vi "Begin.vi"() -> (0 "error out":errorcluster)   [LabVIEW 2014]
doc: "Called before other user functions, this VI is expected to open initial I/O refnums, load in file data, and do all program initialization. Notice that the <B>error out</B> terminal is simply used for data flow. Wiring it to other structures or subVIs ensures that this VI runs first."
uses:
  <vilib>/Rock Robotics/SystemInterfaces/DIO/FPGA_DIOPWMChannel.ctl
  <vilib>/Rock Robotics/WPI/SafetyOutput/WPI_SafetyOutputConfigMenu.ctl
  <vilib>/Rock Robotics/WPI/DriverStation/WPI_DriverStationRobotMode2.ctl
  <vilib>/Rock Robotics/WPI/Joystick/WPI_JoystickDeviceEnum.ctl
  <vilib>/Rock Robotics/SystemInterfaces/AI/FPGA_AIChannel.ctl
  <vilib>/Rock Robotics/SystemInterfaces/AI/FPGA_AIGyroChannel.ctl
  <vilib>/Rock Robotics/SystemInterfaces/DIO/FPGA_DIOChannel.ctl
  <vilib>/Rock Robotics/SystemInterfaces/DIO/FPGA_DIORelayChannel.ctl
  Robot Global Data.vi
  <vilib>/Rock Robotics/WPI/RobotDrive/WPI_RobotDriveOpen4MotorWithVictor.vi
  <vilib>/Rock Robotics/WPI/MotorControl/WPI_MotorControlOpen Victor.vi
  Events.vi
  Robot Global ref.vi
  AutonVars.vi
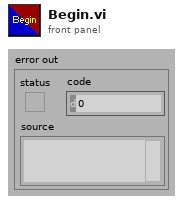
[diagram p1: front panel]
types:
  T1 = typedef "FPGA_DIORelayChannel.ctl" = enum8{"Relay 1", "Relay 2", "Relay 3", "Relay 4", "Relay 5", "Relay 6", "Relay 7", "Relay 8", "Invalid"}
  T2 = typedef "FPGA_DIOChannel.ctl" = enum8{"DIO 1", "DIO 2", "DIO 3", "DIO 4", "DIO 5", "DIO 6", "DIO 7", "DIO 8", "DIO 9", "DIO 10", "DIO 11", "DIO 12", "DIO 13", "DIO 14", "Invalid"}
  T3 = typedef "FPGA_DIOPWMChannel.ctl" = enum8{"PWM 1", "PWM 2", "PWM 3", "PWM 4", "PWM 5", "PWM 6", "PWM 7", "PWM 8", "PWM 9", "PWM 10", "Invalid"}
  T4 = typedef "FPGA_AIGyroChannel.ctl" = enum8{"AI 1", "AI 2", "Invalid"}
  T5 = typedef "WPI_JoystickDeviceEnum.ctl" = enum16{"USB 0", "USB 1", "USB 2", "USB 3", "USB 4", "USB 5"}
  T6 = typedef "FPGA_AIChannel.ctl" = enum8{"AI 1", "AI 2", "AI 3", "AI 4", "AI 5", "AI 6", "AI 7", "AI 8", "Invalid"}
  T7 = typedef "WPI_DriverStationRobotMode2.ctl" = enum16{"Autonomous Disabled", "Autonomous Enabled", "Teleop Disabled", "Teleop Enabled", "Disconnected", "Finish", "Test Disabled", "Test Enabled"}
  T8 = typedef "WPI_SafetyOutputConfigMenu.ctl" = enum16{"Enable", "Disable"}
  T9 = typedef "WPI_RobotDriveDevRef.ctl" = cluster{"DevStatus":errorcluster, "Motors[]":T10[], "Square Inputs":bool, "Max Output":dbl}
  T10 = typedef "WPI_MotorControlDeviceRef.ctl" = cluster{"DeviceStatus":errorcluster, "Type":enum16{"PWM", "CAN"}, "PWM":cluster{"Digital Module":T11, "PWM Channel":T3, "DeadBand":T12}, "CAN":cluster{"Device Number":u8, "Control Mode":T13, "Semaphore":T14, "Max Vout":dbl}, "Invert":bool, "TransformRef":T15, "InvTransformRef":T15}
  T11 = typedef "FPGA_TypedefDigitalModule.ctl" = enum16{"Digital Module 1", "Digital Module 2"}
  T12 = typedef "WPI_PWMDeadband.ctl" = cluster{"Name":string, "maxPositivePwm":i32, "minPositivePwm":i32, "centerPwm":i32, "maxNegativePwm":i32, "minNegativePwm":i32, "angularRange":u16}
  T13 = typedef "WPI_CANJaguar_ControlMode.ctl" = enum8{"Percent VBus", "Current", "Speed", "Position", "Voltage"}
  T14 = typedef "Semaphore RefNum" = refnum<k1>
  T15 = typedef "WPI_PWMTransform_ConPane.ctl" = refnum<vi>
  T16 = typedef "WPI_DigitalInputDevRef.ctl" = cluster{"DevStatus":errorcluster, "DIO Channel":T2, "Digital Module":T11}
  T17 = typedef "WPI_GyroDevRef.ctl" = cluster{"DevStatus":errorcluster, "Analog Module":T18, "Analog Channel":T6, "Offset":dbl, "Gain (VoltsPerDegree/Second)":dbl}
  T18 = typedef "FPGA_TypedefAnalogModule.ctl" = enum16{"Analog Module 1", "Analog Module 2"}
  T19 = typedef "WPI_ServoDeviceRef.ctl" = cluster{"DeviceStatus":errorcluster, "Digital Module":T11, "PWM Channel":T3, "DeadBand":T12}
  T20 = typedef "WPI_JoystickDevRef.ctl" = cluster{"Device":T5}
  T21 = typedef "WPI_AnalogChannelDevRef.ctl" = cluster{"DevStatus":errorcluster, "Analog Module":T18, "Analog Channel":T6}
  T22 = typedef "WPI_RelayDevRef.ctl" = cluster{"DevStatus":errorcluster, "Relay Channel":T1, "Digital Module":T11, "Relay Direction":T23}
  T23 = typedef "WPI_RelayDirection.ctl" = enum16{"Both directions", "Forward only", "Reverse only"}
  T24 = typedef "Eventgrab.ctl" = cluster{"Grab":bool, "GroundPass":bool, "Test Aqaure":dbl, "Shoulder up or down?":bool, "Auton drag":bool}
  T25 = typedef "Robot Global ref.ctl" = cluster{"Joysticks":cluster{"OpJoystickRef":T20, "DriveJoystickRef":T20, "DriveJoystickRef2":T20}, "Drive Motors Ref":cluster{"RobotDriveDevRef":T9}, "Ultrasonic":cluster{"AIDeviceRef":T21}, "Shifters":cluster{"SolenoidDevRef":T26}, "Gyro":cluster{"GyroDevRef":T17}, "Acquistion sensor":cluster{"HighDIO":T16, "Acquisition Bottom1":T16, "Acquisition Top":T16, "Acquisition Bottom2":T16}, "Motors":cluster{"AcqMotorRef":T10, "ShooterMotorRef":T10, "AcqshoulderControlDeviceRef":T10, "LatchControlDeviceRef":T10}, "Servos":cluster{"Winch Servo ":T19, "TrajectorycontrolDeviceRef":T19}, "Shooter Latch Sensors":cluster{"Shooter Latch Sensor Top":T16, "Shooter Latch Sensor Bottom":T16}, "Ring light relay":cluster{"RelayDevRef":T22}}
  T26 = typedef "WPI_SolenoidDevRef.ctl" = cluster{"DevStatus":errorcluster, "Solenoid Module":T27, "Forward Solenoid Channel":T28, "Reverse Solenoid Channel":T28}
  T27 = typedef "FPGA_TypedefSolenoidModule.ctl" = enum16{"Solenoid Module 1", "Solenoid Module 2"}
  T28 = typedef "WPI_SolenoidChannel.ctl" = enum8{"Solenoid 1", "Solenoid 2", "Solenoid 3", "Solenoid 4", "Solenoid 5", "Solenoid 6", "Solenoid 7", "Solenoid 8", "Invalid"}
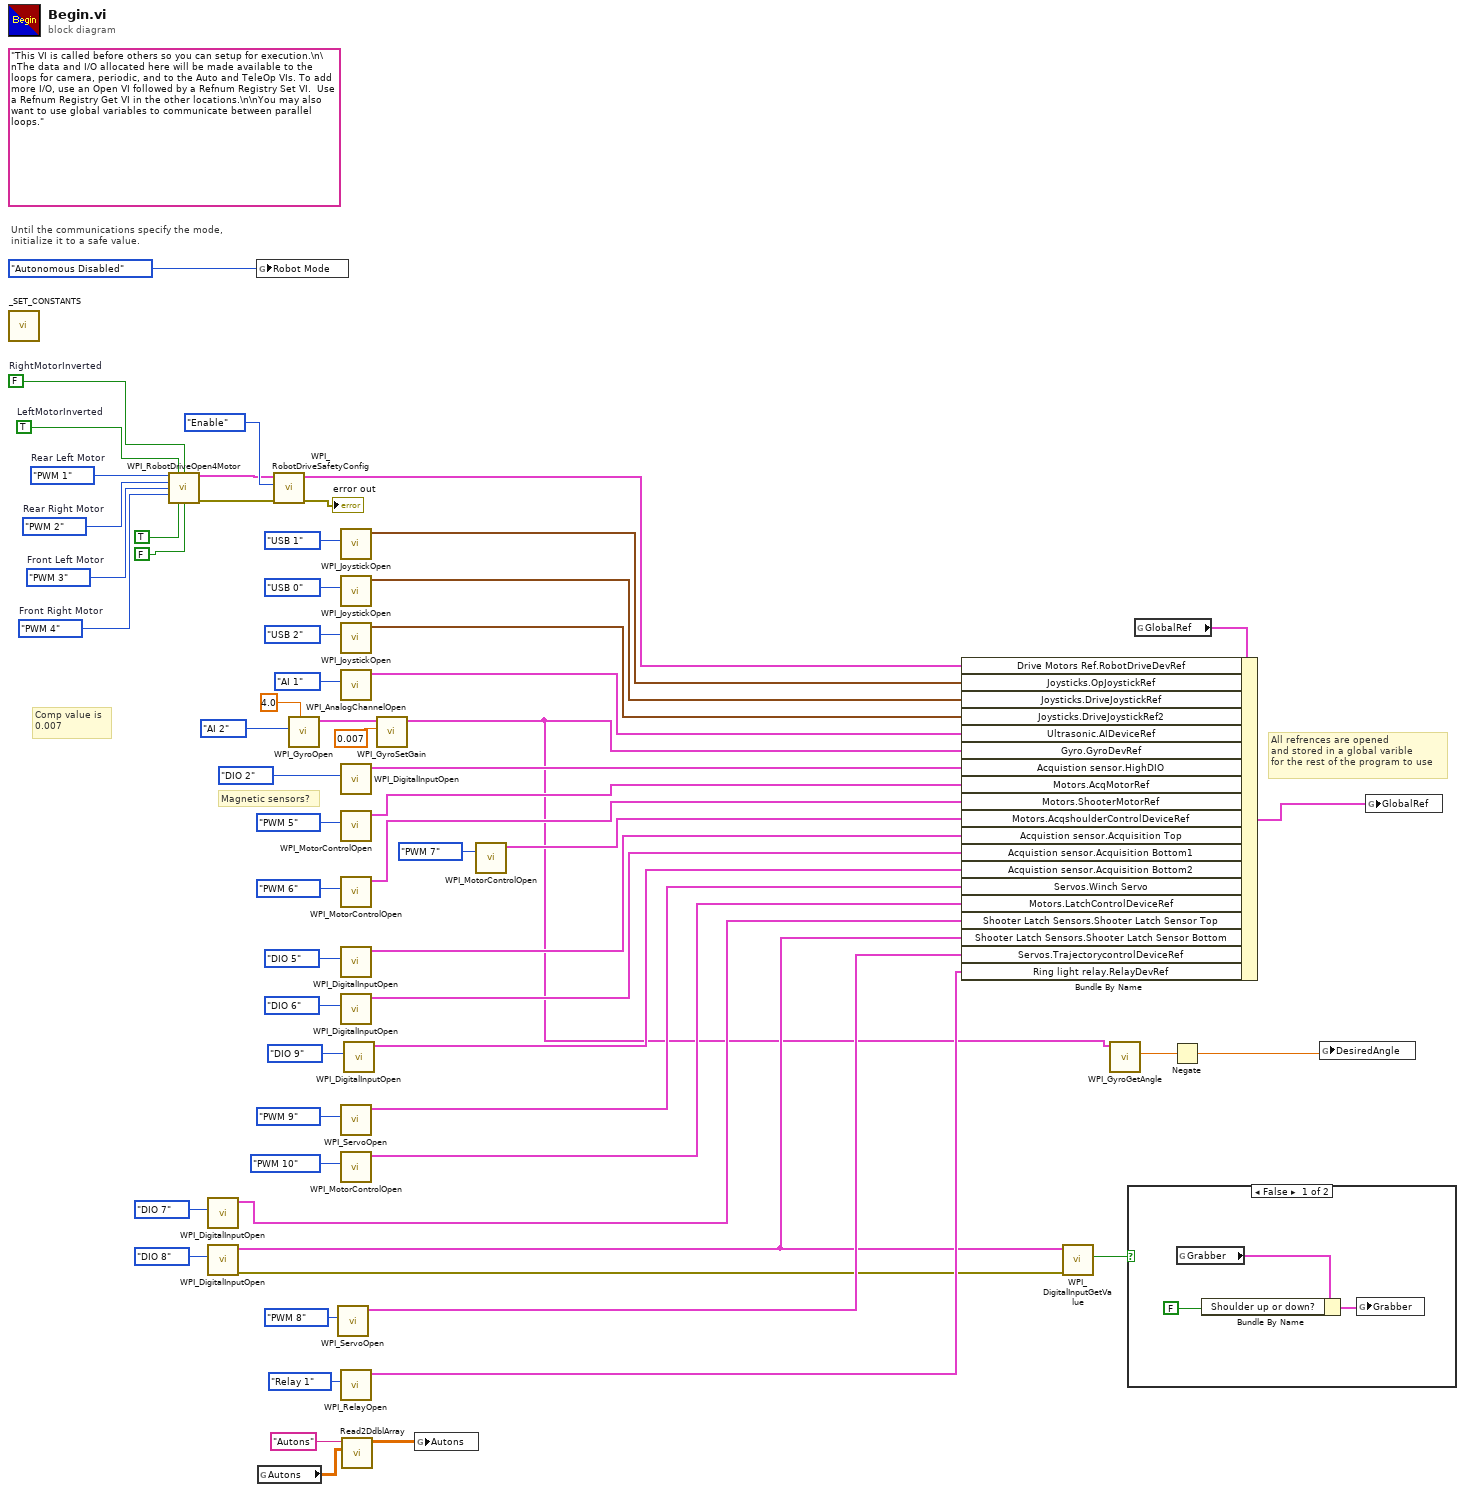
[diagram p0: block diagram]
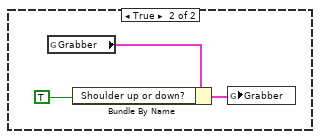
[diagram p2: hidden frame]
diagram:
  w44 = FPGA_DIOPWMChannel."PWM 4"  # Front Right Motor
  w45 = FPGA_DIOPWMChannel."PWM 3"  # Front Left Motor
  (unwired) "This VI is called before others so you can setup for execution.\n\nThe data and I/O allocated here will be made available to the loops for camera, periodic, and to the Auto and TeleOp VIs. To add more I/O, use an Open VI followed by a Refnum Registry Set VI.  Use a Refnum Registry Get VI in the other locations.\n\nYou may also want to use global variables to communicate between parallel loops."
  w59 = FPGA_DIOPWMChannel."PWM 2"  # Rear Right Motor
  w60 = FPGA_DIOPWMChannel."PWM 1"  # Rear Left Motor
  w61 = TRUE  # LeftMotorInverted
  w62 = FALSE  # RightMotorInverted
  # "Comp value is\n0.007"
  # "All refrences are opened \nand stored in a global varible \nfor the rest of the program to use"
  # "Magnetic sensors?"
  # "Until the communications specify the mode,\ninitialize it to a safe value."
  n1 = call "_SET_CONSTANTS.vi"() -> ()  [unwired: 12 in]
  n2 = call-poly <vilib>:"WPI_RobotDriveOpen4Motor.vi"("Rear Left Motor"=w60, "Rear Left Motor Inverted"=w61, "Rear Right Motor Inverted"=w62, "Rear Right Motor"=w59, "Front Left Motor"=w45, "Front Right Motor"=w44, "Front Left Motor Inverted"=TRUE, "Front Right Motor Inverted"=FALSE) -> ("RobotDriveDevRef"=w50:T9, "error out"=w48:errorcluster)  [unwired: 6 in]
  n3 = call <vilib>:"WPI_DigitalInputOpen.vi"("DIO Channel"=FPGA_DIOChannel."DIO 7") -> ("DigitalInputDevRef"=w19:T16)  [unwired: 9 in, 1 out]
  n4 = call <vilib>:"WPI_DigitalInputOpen.vi"("DIO Channel"=FPGA_DIOChannel."DIO 8") -> ("error out"=w10:errorcluster, "DigitalInputDevRef"=w9:T16)  [unwired: 9 in]
  n5 = global write "Robot Global Data.vi" "Robot Mode"(WPI_DriverStationRobotMode2."Autonomous Disabled" ("Robot Mode")) -> ()
  n6 = global read "AutonVars.vi" "Autons"() -> (w5:dbl[][])
  n7 = call <vilib>:"WPI_RobotDriveSafetyConfig.vi"("error in (no error)"=w48, "mode"=WPI_SafetyOutputConfigMenu."Enable", "RobotDriveDevRef"=w50) -> ("error out"=→"error out":errorcluster, "RobotDriveDevRef"=w49:T9)  [unwired: 7 in]
  n8 = call <vilib>:"WPI_GyroOpen.vi"("Calibration Time (s)"=4.0, "Analog Channel"=FPGA_AIGyroChannel."AI 2") -> ("GyroDevRef"=w18:T17)  [unwired: 7 in, 2 out]
  n9 = call <vilib>:"WPI_ServoOpen.vi"("PWM Channel"=FPGA_DIOPWMChannel."PWM 8") -> ("ServoDeviceRef"=w15:T19)  [unwired: 9 in, 1 out]
  n10 = call <vilib>:"WPI_JoystickOpen.vi"("JoystickDevice"=WPI_JoystickDeviceEnum."USB 1") -> ("JoystickDevRef"=w52:T20)  [unwired: 10 in]
  n11 = call <vilib>:"WPI_JoystickOpen.vi"("JoystickDevice"=WPI_JoystickDeviceEnum."USB 0") -> ("JoystickDevRef"=w51:T20)  [unwired: 10 in]
  n12 = call <vilib>:"WPI_JoystickOpen.vi"("JoystickDevice"=WPI_JoystickDeviceEnum."USB 2") -> ("JoystickDevRef"=w39:T20)  [unwired: 10 in]
  n13 = call <vilib>:"WPI_AnalogChannelOpen.vi"("Analog Channel"=FPGA_AIChannel."AI 1") -> ("AIDeviceRef"=w41:T21)  [unwired: 9 in, 1 out]
  n14 = call <vilib>:"WPI_DigitalInputOpen.vi"("DIO Channel"=FPGA_DIOChannel."DIO 2") -> ("DigitalInputDevRef"=w36:T16)  [unwired: 9 in, 1 out]
  n15 = call-poly <vilib>:"WPI_MotorControlOpen.vi"("PWM Channel"=FPGA_DIOPWMChannel."PWM 5") -> ("MotorControlDeviceRef"=w32:T10)  [unwired: 9 in, 1 out]
  n16 = call-poly <vilib>:"WPI_MotorControlOpen.vi"("PWM Channel"=FPGA_DIOPWMChannel."PWM 6") -> ("MotorControlDeviceRef"=w33:T10)  [unwired: 9 in, 1 out]
  n17 = call <vilib>:"WPI_DigitalInputOpen.vi"("DIO Channel"=FPGA_DIOChannel."DIO 5") -> ("DigitalInputDevRef"=w27:T16)  [unwired: 9 in, 1 out]
  n18 = call <vilib>:"WPI_DigitalInputOpen.vi"("DIO Channel"=FPGA_DIOChannel."DIO 6") -> ("DigitalInputDevRef"=w26:T16)  [unwired: 9 in, 1 out]
  n19 = call <vilib>:"WPI_ServoOpen.vi"("PWM Channel"=FPGA_DIOPWMChannel."PWM 9") -> ("ServoDeviceRef"=w25:T19)  [unwired: 9 in, 1 out]
  n20 = call-poly <vilib>:"WPI_MotorControlOpen.vi"("PWM Channel"=FPGA_DIOPWMChannel."PWM 10") -> ("MotorControlDeviceRef"=w22:T10)  [unwired: 9 in, 1 out]
  n21 = call <vilib>:"WPI_RelayOpen.vi"("Relay Channel"=FPGA_DIORelayChannel."Relay 1") -> ("RelayDevRef"=w11:T22)  [unwired: 9 in, 1 out]
  n22 = call "Read2DdblArray.vi"("Default"=w5, "Name"="Autons") -> ("Read"=w7:dbl[][])  [unwired: 9 in]
  n23 = call <vilib>:"WPI_DigitalInputOpen.vi"("DIO Channel"=FPGA_DIOChannel."DIO 9") -> ("DigitalInputDevRef"=w12:T16)  [unwired: 9 in, 1 out]
  n24 = call <vilib>:"WPI_GyroSetGain.vi"("Gain (VoltsPerDegree/Second)"=0.007, "GyroDevRef"=w18) -> ("GyroDevRef"=w3:T17)  [unwired: 8 in, 1 out]
  n25 = global write "AutonVars.vi" "Autons"(w7) -> ()
  n26 = call-poly <vilib>:"WPI_MotorControlOpen.vi"("PWM Channel"=FPGA_DIOPWMChannel."PWM 7") -> ("MotorControlDeviceRef"=w30:T10)  [unwired: 9 in, 1 out]
  n27 = call <vilib>:"WPI_DigitalInputGetValue.vi"("error in (no error)"=w10, "DigitalInputDevRef"=w9) -> ("Value"=w8:bool)  [unwired: 7 in, 2 out]
  n28 = call <vilib>:"WPI_GyroGetAngle.vi"("GyroDevRef"=w3) -> ("Angle"=w2:dbl)  [unwired: 7 in, 3 out]
  n29 = case shown="False" w8 {
    frame False {
      n30 = global read "Events.vi" "Grabber"() -> (w65:T24)
      n31 = Bundle By Name(cluster=w65, "Shoulder up or down?"=FALSE) -> (w63:T24)
      n32 = global write "Events.vi" "Grabber"(w63) -> ()
    }
    frame True {
      n33 = global read "Events.vi" "Grabber"() -> (w68:T24)
      n34 = Bundle By Name(cluster=w68, "Shoulder up or down?"=TRUE) -> (w66:T24)
      n35 = global write "Events.vi" "Grabber"(w66) -> ()
    }
  }
  n36 = global read "Robot Global ref.vi" "GlobalRef"() -> (w53:T25)
  n37 = Bundle By Name(cluster=w53, "Drive Motors Ref.RobotDriveDevRef"=w49, "Joysticks.OpJoystickRef"=w52, "Joysticks.DriveJoystickRef"=w51, "Joysticks.DriveJoystickRef2"=w39, "Ultrasonic.AIDeviceRef"=w41, "Gyro.GyroDevRef"=w3, "Acquistion sensor.HighDIO"=w36, "Motors.AcqMotorRef"=w32, "Motors.ShooterMotorRef"=w33, "Motors.AcqshoulderControlDeviceRef"=w30, "Acquistion sensor.Acquisition Top"=w27, "Acquistion sensor.Acquisition Bottom1"=w26, "Acquistion sensor.Acquisition Bottom2"=w12, "Servos.Winch Servo"=w25, "Motors.LatchControlDeviceRef"=w22, "Shooter Latch Sensors.Shooter Latch Sensor Top"=w19, "Shooter Latch Sensors.Shooter Latch Sensor Bottom"=w9, "Servos.TrajectorycontrolDeviceRef"=w15, "Ring light relay.RelayDevRef"=w11) -> (w54:T25)
  n38 = Negate(x=w2) -> (-x=w1:dbl)
  n39 = global write "Events.vi" "DesiredAngle"(w1) -> ()
  n40 = global write "Robot Global ref.vi" "GlobalRef"(w54) -> ()
